vi "RSNRPZ Set Trigger Synchronization State.vi"(8 "error in (no error)":errorcluster, 9 "State (F: Off)":bool, 10 "Channel (1)":i32=1, 11 "VISA session":refnum<visa-resource-name> caption="VISA resource name") -> (0 "error out":errorcluster, 3 "dup VISA session":refnum<visa-resource-name> caption="VISA resource name")   [LabVIEW 2010]
doc: "This VI can be used to synchronize the sensors connected to the trigger bus. Synchronization is achieved by enabling the\ntrigger signal only when all the sensors are in the WAIT_FOR_TRIGGER state (wired-OR). This ensures that the measurements are started simultaneously and also that repetitions due to averaging start at the same time. It must be ensured that the number of repetitions is the same for all the sensors involved in the measurement. Otherwise, the trigger bus will be blocked by any sensor that has completed its measurements before the others and has returned to the IDLE state.\n\nRemote-control command(s):\nTRIG:SYNC:STAT ON | OFF"
uses:
  rsnrpz_32.dll
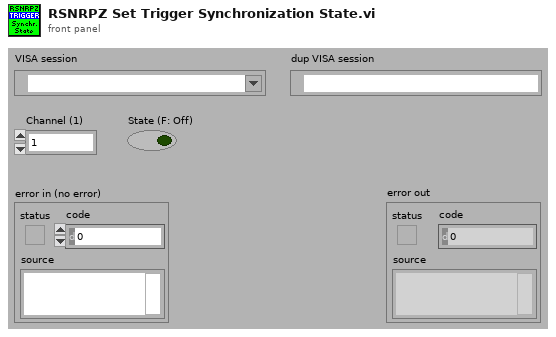
[diagram p1: front panel]
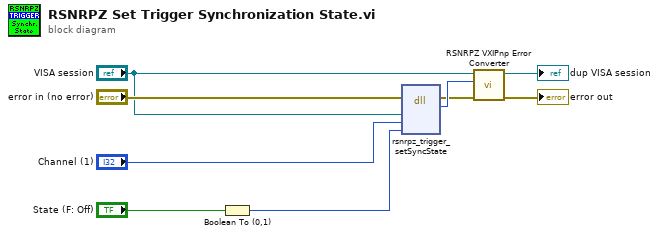
[diagram p0: block diagram]
diagram:
  n1 = Boolean To (0,1)(Boolean="State (F: Off)") -> (0, 1=w6:i16)
  n2 = dll-call lib="rsnrpz_32.dll" fn="rsnrpz_trigger_setSyncState"(error in="error in (no error)", "Instrument Handle"="VISA session", "Channel"="Channel (1)", "State"=w6) -> (error out=w5:errorcluster, "Status"=w8:i32)  [unwired: 5 in, 1 out]
  n3 = call <instrlib>:"RSNRPZ VXIPnp Error Converter.vi"("error in"=w5, "VXIPnp error code"=w8, "VISA session"="VISA session") -> ("error out"=→"error out":errorcluster, "dup VISA session"=→"dup VISA session":refnum<visa-resource-name>)  [unwired: 7 in]
